vi "VescSetRpm.vi"(10 "error in (no error)":errorcluster, 11 "Speed (rpm)":i32) -> (2 "error out":errorcluster)   [LabVIEW 2019]
uses:
  <vilib>/myRIO/Instrument Drivers/Onboard IO/UART/typedef/VISA Configuration.ctl
  <vilib>/Instr/_visa.llb/VISA Configure Serial Port (Instr).vi
  <vilib>/myRIO/Express VI/Onboard IO/UART/UART Express VI.xnode
  <vilib>/myRIO/Instrument Drivers/Onboard IO/UART/UART.lvlib
  Downloads/libvesc.so
panel:
  in  "stop":bool
  out "Read VESC":u8[](array[numeric])
  out "Read":string
  out "OutputFromC":u8[](array[numeric])
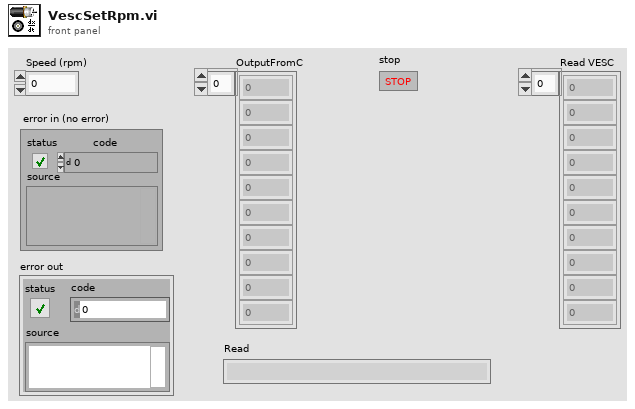
[diagram p1: front panel]
types:
  T1 = typedef "UART.lvlib/VISA Configuration.ctl" = cluster{"baud rate (9600)":u32, "data bits (8)":u16, "parity (0:none)":enum16{"None", "Odd", "Even", "Mark", "Space"}, "stop bits (10: 1 bit)":u16, "flow control (0:none)":u16, "termination char\n(0xA = '\\n' = LF) ":u8, "Enable Termination\nChar (T)":bool, "timeout (10sec)":u32}
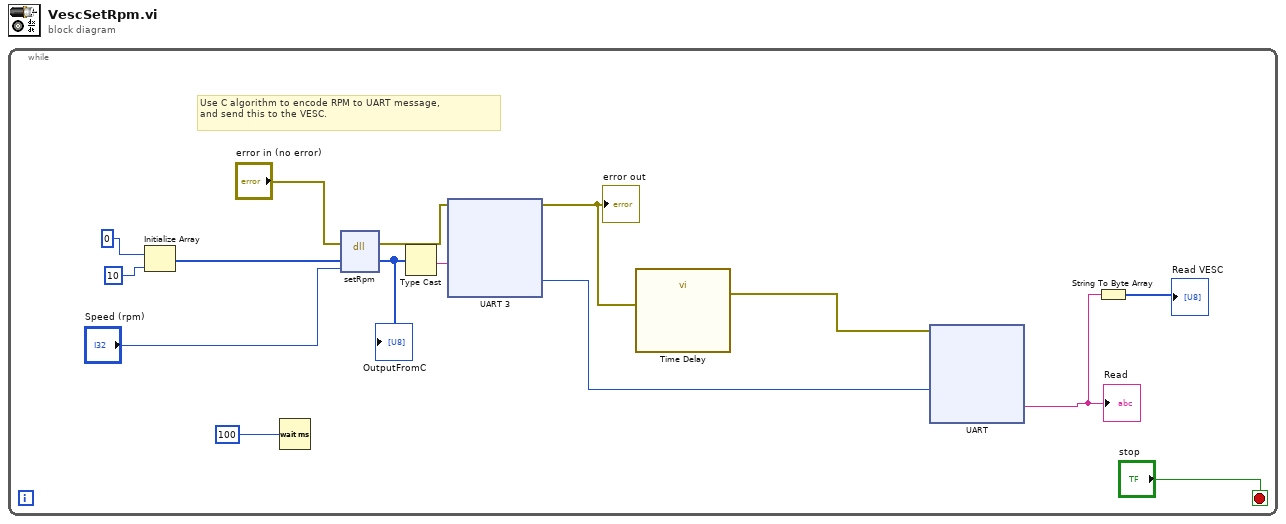
[diagram p0: block diagram]
diagram:
  n1 = while {
    stop <- "stop" stop-if-true
    # "Use C algorithm to encode RPM to UART message,\nand send this to the VESC."
    n2 = Initialize Array(0, 10) -> (w9:i32[])
    n3 = Wait (ms)(milliseconds to wait=100) -> ()  [unwired: 1 out]
    n4 = dll-call lib="C:/Users/Joakim Nylander N/Downloads/libvesc.so" fn="setRpm"(error in="error in (no error)", "array"=w9, "rpm"="Speed (rpm)") -> (error out=w8:errorcluster, "array"=w5:u8[])  [unwired: 4 in, 1 out]
    "OutputFromC" <- w5
    n5 = Type Cast(x=w5) -> (*(type *) &x=w6:string)  [unwired: 1 in]
    n6 = xnode "UART 3"("Characters to Write"=w6, "error in (no error)"=w8) -> ("Character Count"=w12:u32, "error out"=w13:errorcluster)
    "error out" <- w13
    n7 = call "Time Delay"("error in (no error)"=w13) -> ("error out"=w11:errorcluster)  [unwired: 10 in]
    n8 = xnode "UART"("Character Count"=w12, "error in (no error)"=w11) -> ("Characters Read"=w14:string)  [unwired: 1 out]
    "Read" <- w14
    n9 = String To Byte Array(string=w14) -> (unsigned byte array=→"Read VESC":u8[])
  }
